vi "Get Experiments.vi"(3 "error in (no error)":errorcluster, 5 "Database.lvlib:Data Store.lvclass":refnum<class "Data Store.lvclass">) -> (0 "error out":errorcluster, 1 "Array":T1[](array[typedef]), 2 "Database.lvlib:Data Store.lvclass 2":refnum<class "Data Store.lvclass">)   [LabVIEW 2012, in "Database.lvlib" / "Data Store.lvclass"]
uses:
  Data Store.lvclass
  Experiment.ctl
  Data Store.lvclass/Data Store.ctl
  <vilib>/addons/database/_DB Variant To Data/Database Variant To Data.xnode
  <vilib>/addons/database/NI_Database_API.lvlib
  Database.lvlib
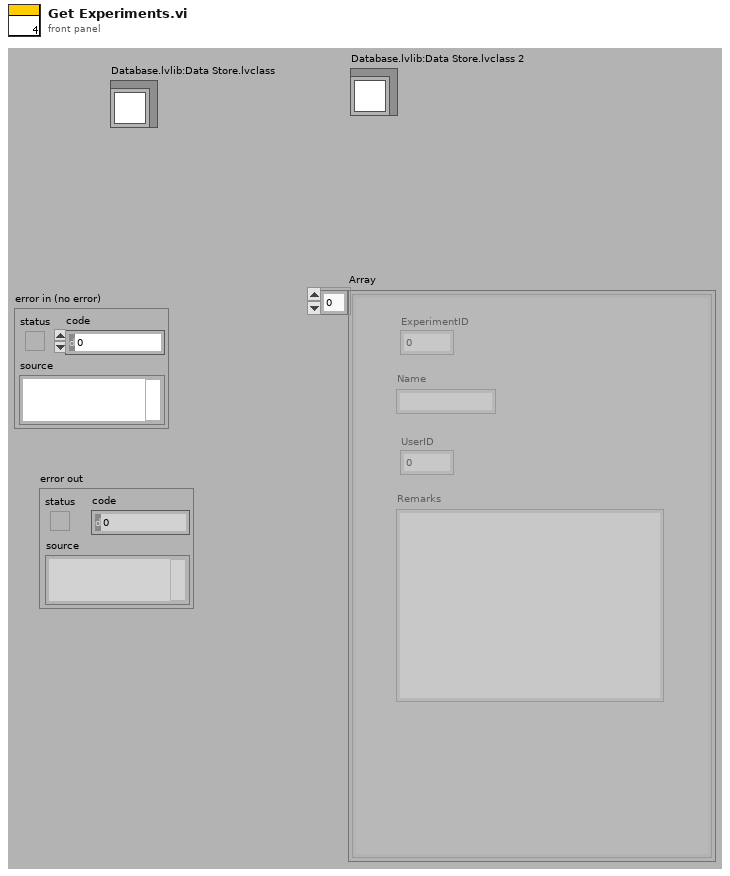
[diagram p1: front panel]
types:
  T1 = typedef "Database.lvlib/Experiment.ctl" = cluster{"ExperimentID":i32, "Name":string, "UserID":i32, "Remarks":string}
  T2 = typedef "NI_Database_API.lvlib/Conn ObjectReference.ctl" = refnum<k1>
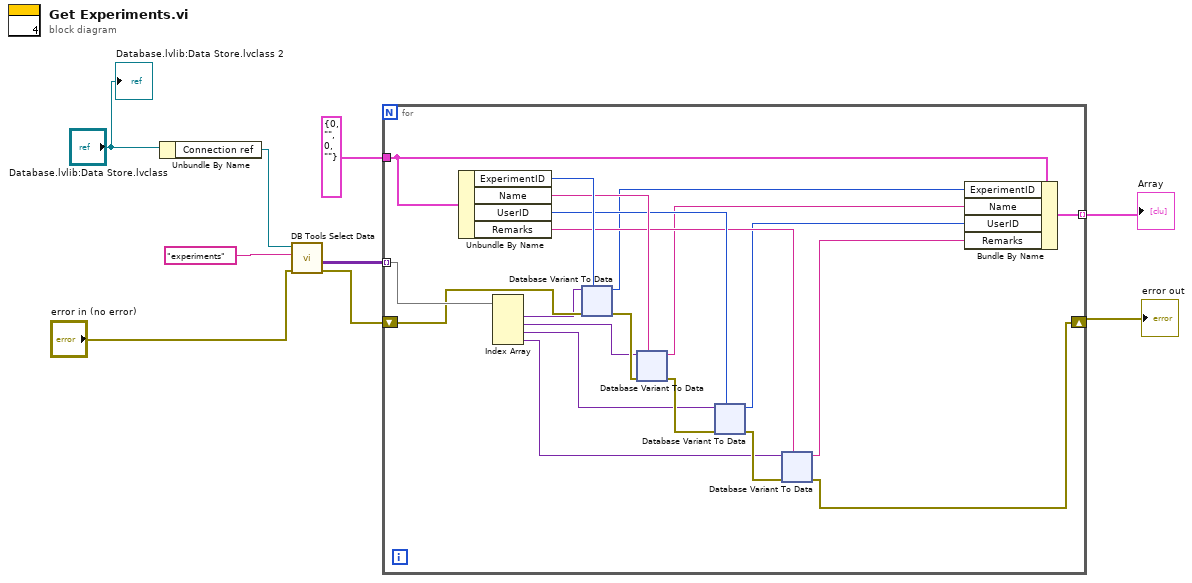
[diagram p0: block diagram]
diagram:
  n1 = Unbundle By Name("Database.lvlib:Data Store.lvclass") -> ("Connection ref"=w9:T2)
  n2 = call <vilib>:"DB Tools Select Data.vi"("error in (no error)"="error in (no error)", "table"="experiments", "connection reference"=w9) -> ("error out"=w5:errorcluster, "data"=w4:variant[][])  [unwired: 3 in, 1 out]
  n3 = for {
    tunnel: w4 -> [w29] mode=indexing
    tunnel: T1 {"ExperimentID"=0, "Name"="", "UserID"=0, "Remarks"=""} ("Cluster") -> [w23]
    shift-right: [w10] -> w1
    shift-left: w5 -> [w28]
    tunnel: [w14] -> w2 mode=indexing
    n4 = Unbundle By Name(w23) -> ("ExperimentID"=w22:i32, "Name"=w21:string, "UserID"=w20:i32, "Remarks"=w19:string)
    n5 = Index Array(array=w29) -> (element #1=w24:variant, element #2=w13:variant, element #3=w12:variant, element #4=w11:variant)  [unwired: 4 in]
    n6 = xnode "Database Variant To Data"("database variant"=w24, "error in"=w28, "type"=w22) -> ("data"=w18:i32, "error out"=w27:errorcluster)
    n7 = xnode "Database Variant To Data"("database variant"=w13, "error in"=w27, "type"=w21) -> ("data"=w17:string, "error out"=w26:errorcluster)
    n8 = xnode "Database Variant To Data"("database variant"=w12, "error in"=w26, "type"=w20) -> ("data"=w16:i32, "error out"=w25:errorcluster)
    n9 = xnode "Database Variant To Data"("database variant"=w11, "error in"=w25, "type"=w19) -> ("data"=w15:string, "error out"=w10:errorcluster)
    n10 = Bundle By Name(cluster=w23, "ExperimentID"=w18, "Name"=w17, "UserID"=w16, "Remarks"=w15) -> (w14:T1)
  }
  "error out" <- w1
  "Array" <- w2
  "Database.lvlib:Data Store.lvclass 2" <- "Database.lvlib:Data Store.lvclass"
